vi "ActReadTrajectoryFile.vi"(9 "Index 1,2,3,4":i32, 11 "FileName":string="ThreeBallTrajOne.csv") -> ()   [LabVIEW 2023]
uses:
  <vilib>/Rock Robotics/WPI/ThirdParty/JAS_Junk/TrajLib/Trajectory_Library.lvlib
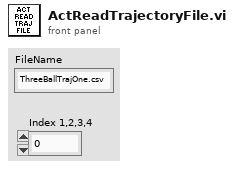
[diagram p1: front panel]
types:
  T1 = typedef "Trajectory_Library.lvlib/TRAJECTORY.ctl" = cluster{"TotalTImeSecs":dbl, "States":T2[]}
  T2 = typedef "Trajectory_Library.lvlib/TRAJ_STATE.ctl" = cluster{"TimeSeconds":dbl, "Velocity":dbl, "Acceleration":dbl, "POSE":T3, "Curvature":dbl}
  T3 = typedef "Trajectory_Library.lvlib/POSE2D.ctl" = cluster{"TRANSLATION":T4, "ROTATION":T5}
  T4 = typedef "Trajectory_Library.lvlib/TRANSLATION2D.ctl" = cluster{"X":dbl, "Y":dbl}
  T5 = typedef "Trajectory_Library.lvlib/ROTATION2D.ctl" = cluster{"VALUE":dbl, "COS":dbl, "SIN":dbl}
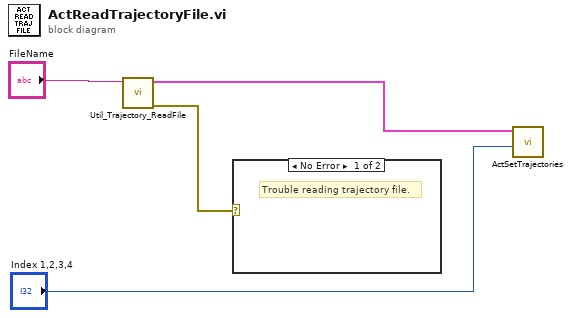
[diagram p0: block diagram]
diagram:
  n1 = call <vilib>:"Util_Trajectory_ReadFile.vi"("FileName"="FileName") -> ("error out"=w4:errorcluster, "outTRAJECTORY"=w1:T1)  [unwired: 8 in, 1 out]
  n2 = case shown="No Error" w4 {
    frame No Error {
      # "Trouble reading trajectory file."
    }
    frame Error {
    }
  }
  n3 = call "ActSetTrajectories.vi"("Index 1,2,3,4"="Index 1,2,3,4", "Trajectory"=w1) -> ()  [unwired: 10 in]
